vi "Sampling Config.vi"(8 "error in (no error)":errorcluster, 11 "Task In":refnum<class "Task Config.lvclass">) -> (0 "error out":errorcluster, 2 "Sampling Config":T1, 3 "Task":refnum<class "Task Config.lvclass">)   [LabVIEW 2020, in "VolatusDAQConfig.lvlib"]
uses:
  VolatusDAQConfig.lvlib
  VolatusConfig/Task/Task Config.lvclass
  C:/dev/lv20CE/relink/lv-volatus/VolatusConfig/VolatusConfigElement/VolatusConfigElement.lvclass
  Sampling Config.ctl
  VolatusConfig/VolatusConfigElement/VolatusConfigElement.lvclass/VolatusConfigElement.ctl
  VolatusConfig/VolatusConfigElement/Element.vi
  VolatusConfig/VolatusConfigElement/VolatusConfigElement.lvclass
  lv-cdm/CDM-Config/Config Element/Config Element.lvclass
  C:/dev/lv20CE/relink/lv-volatus/VolatusConfig/Task/Task Config.lvclass
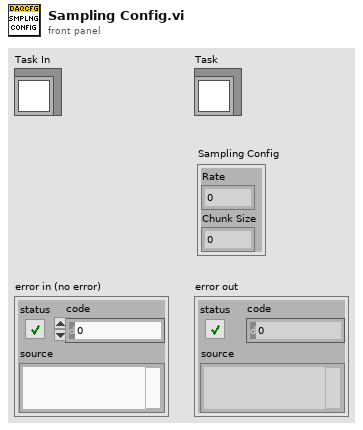
[diagram p1: front panel]
types:
  T1 = typedef "VolatusDAQConfig.lvlib/Sampling Config.ctl" = cluster{"Rate":dbl, "Chunk Size":i32}
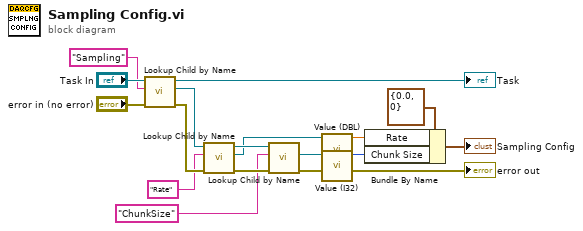
[diagram p0: block diagram]
diagram:
  n1 = call "Lookup Child by Name.vi"("error in (no error)"="error in (no error)", "Child Name"="Sampling", "VolatusConfigElement in"="Task In") -> ("error out"=w17:errorcluster, "Child"=w13:refnum<class "Config Element.lvclass">, "VolatusConfigElement out"=→"Task":refnum<class "Task Config.lvclass">)  [unwired: 5 in, 1 out]
  n2 = call "Lookup Child by Name.vi"("error in (no error)"=w17, "Name"="Rate", "Config Element in"=w13) -> ("error out"=w10:errorcluster, "Child"=w8:refnum<class "Config Element.lvclass">, "Config Element out"=w11:refnum<class "Config Element.lvclass">)  [unwired: 5 in, 1 out]
  n3 = call "Lookup Child by Name.vi"("error in (no error)"=w10, "Name"="ChunkSize", "Config Element in"=w11) -> ("error out"=→"error out":errorcluster, "Child"=w7:refnum<class "Config Element.lvclass">)  [unwired: 5 in, 2 out]
  n4 = call "Value (DBL).vi"("Config Element in"=w8) -> ("DBL Value"=w5:dbl)  [unwired: 9 in, 1 out]
  n5 = call "Value (I32).vi"("Config Element in"=w7) -> ("I32 Value"=w4:i32)  [unwired: 9 in, 1 out]
  n6 = Bundle By Name(cluster=T1 {"Rate"=0.0, "Chunk Size"=0} ("Sampling Config"), "Rate"=w5, "Chunk Size"=w4) -> (→"Sampling Config":T1)
